vi "Main_Robot_Control.vi"() -> ()   [LabVIEW 2014]
uses:
  <instrlib>/Hokuyo URG Series/Public/Initialize-Standard.vi
  <instrlib>/Hokuyo URG Series/Hokuyo URG Series.lvlib
panel:
  in  "polar attributes (hidden)":T1={"maximum"=30000.0, "minimum"=0.0, "clip to min"=FALSE, "log?(F)"=TRUE, "grid color"=6710886, "plot color"=65280, "fmt and prec"={"format"=enum."Decimal", "precision"=0}, "visible section"=8} {"minimum" format="%0.2f"; "maximum" format="%0.2f"}
  in  "Tab Control":T2(tab)
  out "Data Aquired":picture
  out "Blinky LIDAR  Running":bool
  in  "VISA resource name":refnum<visa-resource-name>="COM3"
  in  "Encoding Width":u16(ring)=3 items=["2 Byte"=2, "3 Byte"=3]
  in  "Cluster Count":dbl=1.0
  in  "Start Point":dbl=-50.0
  in  "End Point":dbl=33.0
  in  "Max (m)":dbl=1.0
  in  "Plot Color":u32(colorbox)=14422272
  in  "Grid Color":u32(colorbox)=11776947
  in  "Stop":bool
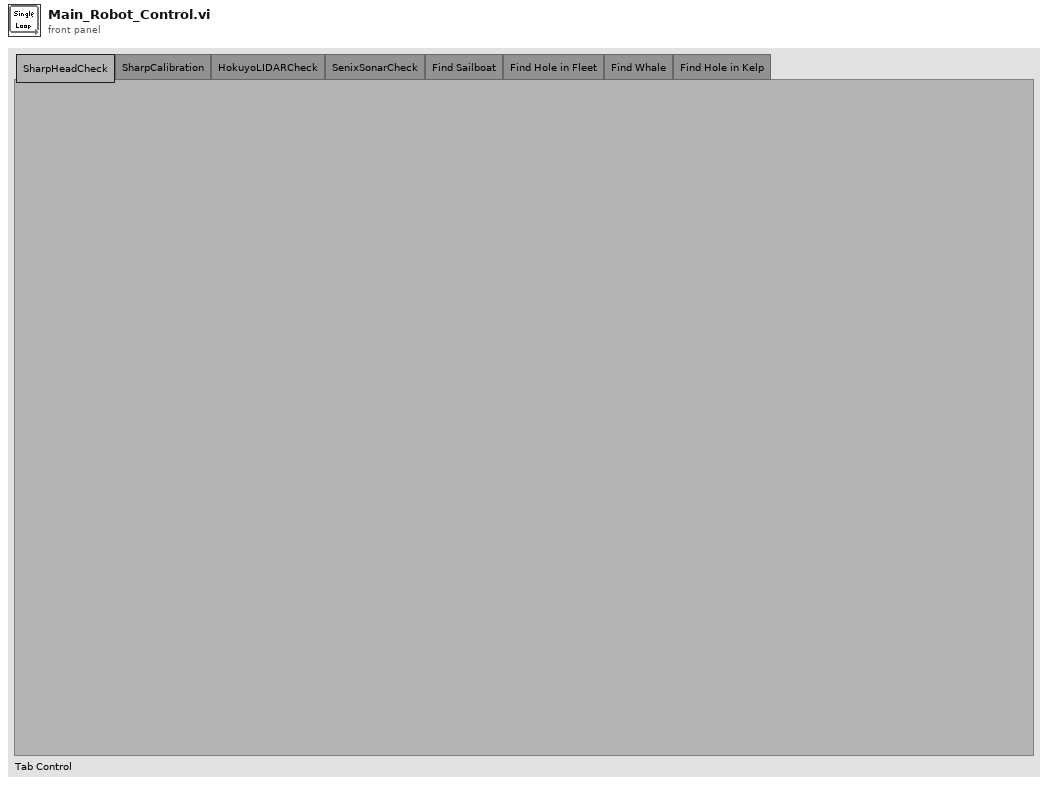
[diagram p1: front panel]
types:
  T1 = cluster{"maximum":dbl, "minimum":dbl, "clip to min":bool, "log?(F)":bool, "grid color":u32, "plot color":u32, "fmt and prec":cluster{"format":enum8{"Decimal", "Scientific", "Engineering", "Binary", "Octal", "Hex"}, "precision":u8}, "visible section":u16}
  T2 = enum32{"SharpHeadCheck", "SharpCalibration", "HokuyoLIDARCheck", "SenixSonarCheck", "Find Sailboat", "Find Hole in Fleet", "Find Whale", "Find Hole in Kelp"}
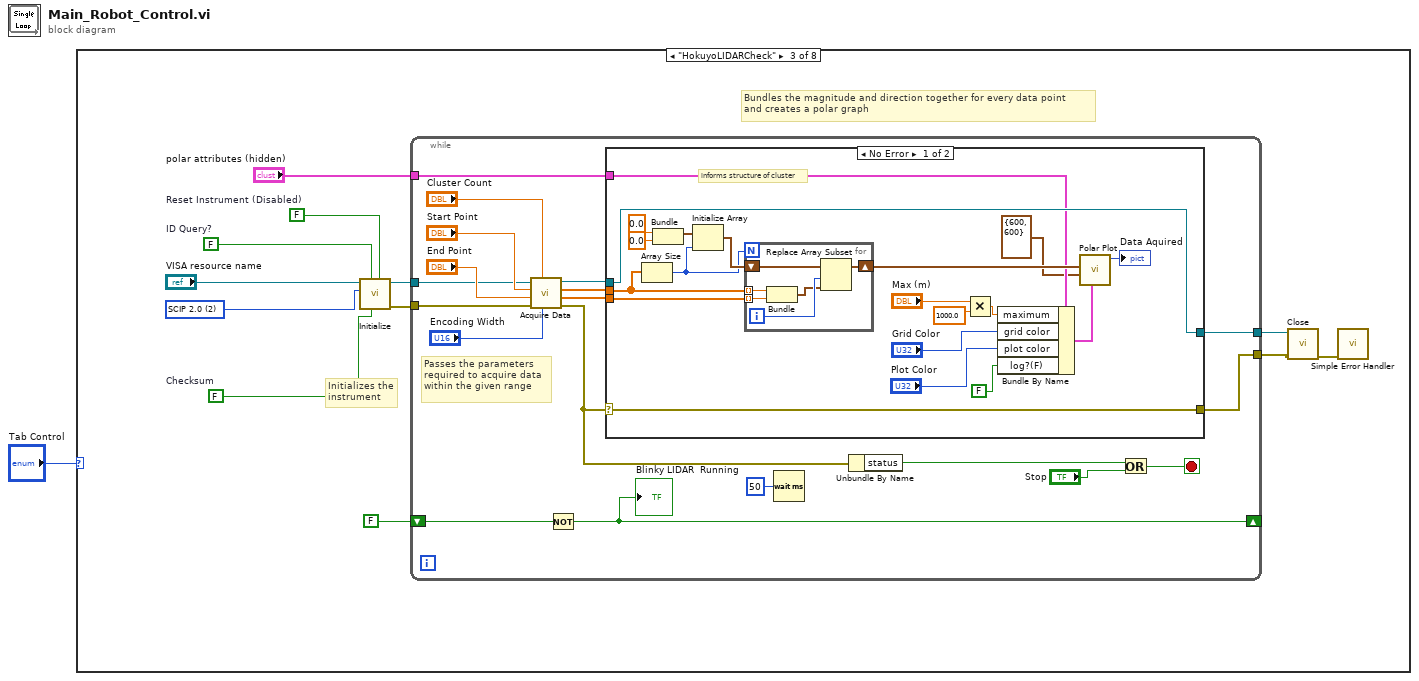
[diagram p0: block diagram]
diagram:
  n1 = case shown="\"HokuyoLIDARCheck\"" "Tab Control" {
    frame "SharpHeadCheck", Default {
    }
    frame "SharpCalibration" {
    }
    frame "HokuyoLIDARCheck" {
      w11 = FALSE  # Checksum
      w9 = FALSE  # ID Query?
      w7 = u32 2 items=["Convert to Latest", "SCIP 1.1", "SCIP 2.0"] ("Protocol")
      w8 = FALSE  # Reset Instrument (Disabled)
      # "Bundles the magnitude and direction together for every data point\nand creates a polar graph"
      # "Initializes the instrument"
      n2 = call-poly <instrlib>:"Initialize.vi"("Reset? (F: No)"=w8, "Checksum (Disabled)"=w11, "ID Query? (Enabled)"=w9, "Protocol (2: SCIP 2.0)"=w7, "VISA resource name"="VISA resource name") -> ("error out"=w4:errorcluster, "VISA resource name out"=w5:refnum<visa-resource-name>)  [unwired: 5 in]
      n3 = while {
        tunnel: w5 -> [w20]
        tunnel: [w32] -> w13
        tunnel: [w31] -> w6
        tunnel: w4 -> [w19]
        tunnel: "polar attributes (hidden)" -> [w18]
        shift-right: [w14] -> _
        shift-left: FALSE -> [w15]
        stop <- w28 stop-if-true
        # "Passes the parameters\nrequired to acquire data\nwithin the given range"
        n4 = call <instrlib>:"Acquire Data.vi"("Data Encoding Width (3 Byte)"="Encoding Width", "Cluster Count (1)"="Cluster Count", "error in (no error)"=w19, "End Point (120°)"="End Point", "Start Point (-120°)"="Start Point", "VISA resource name"=w20) -> ("error out"=w24:errorcluster, "Direction"=w25:dbl[], "Magnitude"=w26:dbl[], "VISA resource name out"=w27:refnum<visa-resource-name>)  [unwired: 2 in]
        n5 = Not(x=w15) -> (.not. x?=w14:bool)
        "Blinky LIDAR  Running" <- w14
        n6 = case shown="No Error" w24 {
          selector: w24 -> [w50 w60]
          tunnel: [w50 w60] -> w32
          tunnel: w27 -> [w51 w59]
          tunnel: [w51 w59] -> w31
          tunnel: w26 -> [w45 _]
          tunnel: w25 -> [w44 _]
          tunnel: w18 -> [w40 _]
          frame No Error {
            # "informs structure of cluster"
            n7 = Array Size(array=w45) -> (size(s)=w43:i32)
            n8 = Bundle(0.0, 0.0) -> (w47:cluster{dbl, dbl})  [unwired: 1 in]
            n9 = Initialize Array(w47, w43) -> (w46:cluster{dbl, dbl}[])
            n10 = for {
              N: w43 -> [_]
              shift-right: [w54] -> w42
              shift-left: w46 -> [w55]
              tunnel: w45 -> [w58] mode=indexing
              tunnel: w44 -> [w57] mode=indexing
              i -> [w56]
              n11 = Bundle(w58, w57) -> (w53:cluster{dbl, dbl})  [unwired: 1 in]
              n12 = Replace Array Subset(array=w55, new element=w53, index=w56) -> (w54:cluster{dbl, dbl}[])
            }
            n13 = Multiply(x="Max (m)", y=1000.0) -> (x*y=w36:dbl)
            n14 = Bundle By Name(cluster=w40, "maximum"=w36, "grid color"="Grid Color", "plot color"="Plot Color", "log?(F)"=FALSE) -> (w41:T1)
            n15 = call <vilib>:"Polar Plot.vi"("polar attributes"=w41, "dimensions (w,h)"=cluster{"width":i16, "height":i16} {"width"=600, "height"=600}, "data array [mag, phase (deg)]"=w42) -> ("new picture"=→"Data Aquired":picture)  [unwired: 8 in]
          }
          frame Error {
          }
        }
        n16 = Wait (ms)(milliseconds to wait=u32 50) -> ()  [unwired: 1 out]
        n17 = Unbundle By Name(w24) -> ("status"=w30:bool)
        n18 = Or(x=w30, y="Stop") -> (x .or. y?=w28:bool)
      }
      n19 = call <instrlib>:"Close.vi"("error in (no error)"=w13, "VISA resource name"=w6) -> ("error out"=w10:errorcluster)  [unwired: 9 in]
      n20 = call <vilib>:"Simple Error Handler.vi"("error in (no error)"=w10) -> ()  [unwired: 4 in, 5 out]
    }
    frame "SenixSonarCheck" {
    }
    frame "Find Sailboat" {
    }
    frame "Find Hole in Fleet" {
    }
    frame "Find Whale" {
    }
    frame "Find Hole in Kelp" {
    }
  }
